vi "Day 24-Decomposed Instructions.vi"() -> ()   [LabVIEW 2021]
panel:
  out "Numeric":u64
  out "Model Number":u64
  in  "Input File":enum32{"example input", "input"}(radio)
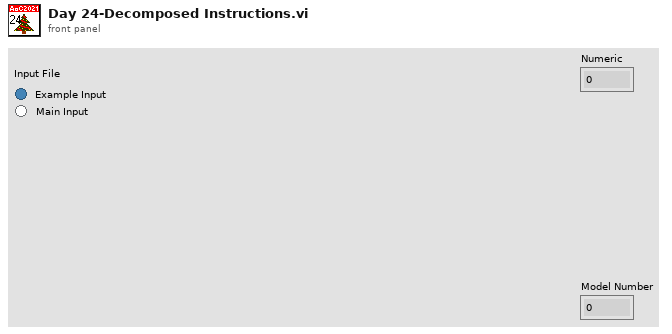
[diagram p1: front panel]
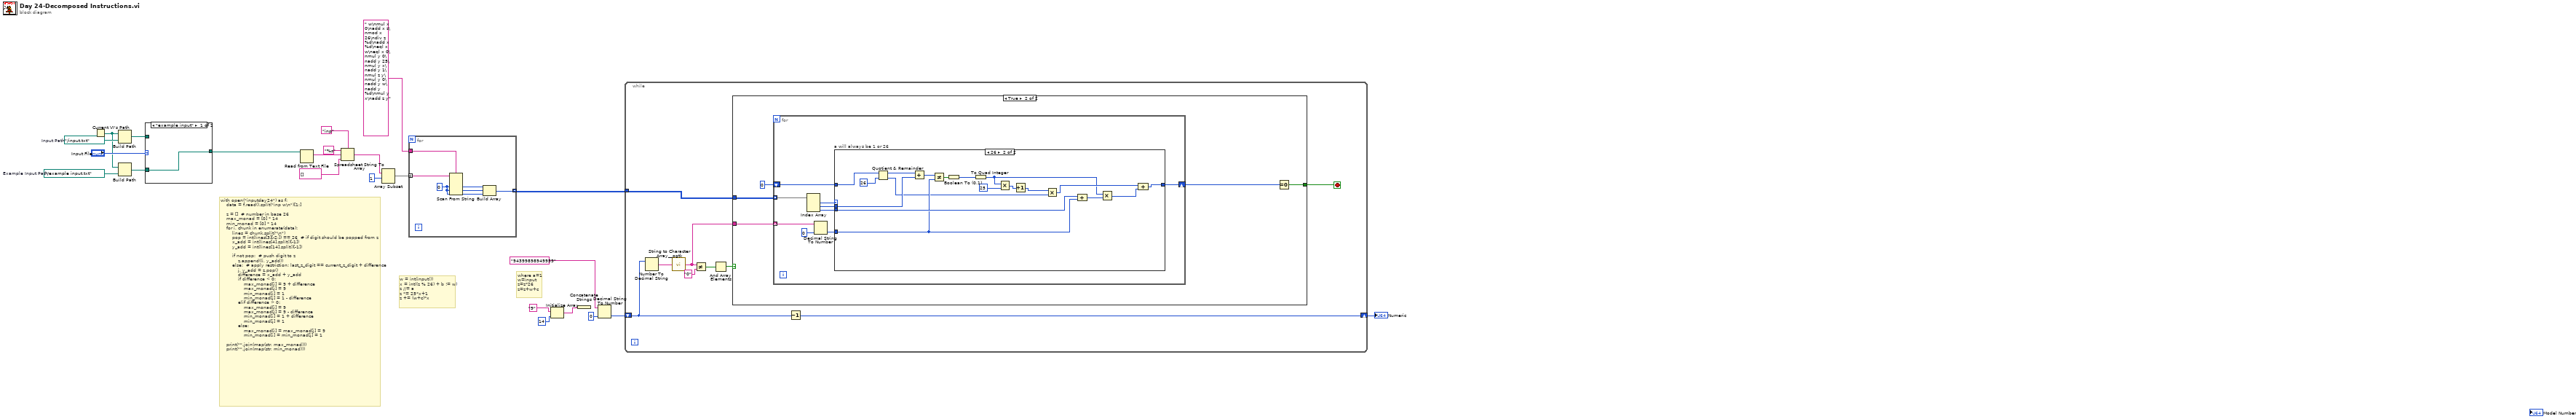
[diagram p0: block diagram]
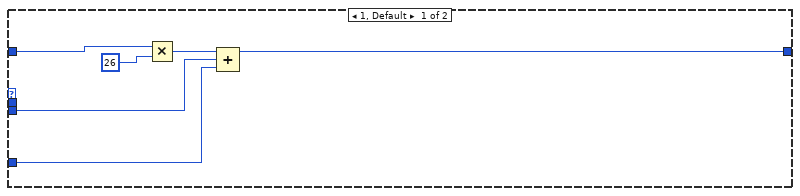
[diagram p4: hidden frame]
diagram:
  w22 = path "../example input.txt"  # Example Input Path
  w23 = path "../input.txt"  # Input Path
  # "with open(\"inputday24\") as f:\n    data = f.read().split(\"inp w\\n\")[1:]\n\n    z = []  # number in base 26\n    max_monad = [0] * 14\n    min_monad = [0] * 14\n    for i, chunk in enumerate(data):\n        lines = chunk.split(\"\\n\")\n        pop = int(lines[3][-2:]) == 26  # if digit should be popped from z\n        x_add = int(lines[4].split()[-1])\n        y_add = int(lines[14].split()[-1])\n\n        if not pop:  # push digit to z\n            z.append((i, y_add))\n        else:  # apply restriction: last_z_digit == current_z_digit + difference\n            j, y_add = z.pop()\n            difference = x_add + y_add\n            if difference < 0:\n                max_monad[i] = 9 + difference\n                max_monad[j] = 9\n                min_monad[i] = 1\n                min_monad[j] = 1 - difference\n            elif difference > 0:\n                max_monad[i] = 9\n                max_monad[j] = 9 - difference\n                min_monad[i] = 1 + difference\n                min_monad[j] = 1\n            else:\n                max_monad[i] = max_monad[j] = 9\n                min_monad[i] = min_monad[j] = 1\n\n    print(\"\".join(map(str, max_monad)))\n    print(\"\".join(map(str, min_monad)))"
  # "w = int(input())\nx = int((z % 26) + b != w)\nz //= a\nz *= 25*x+1\nz += (w+c)*x"
  # "where a=1\nw=input\nz=z*26\nz=z+w+c"
  n1 = Current VI's Path() -> (path=w18:path)
  n2 = Build Path(base path=w18, name or relative path=w23) -> (appended path=w20:path)
  n3 = Build Path(base path=w18, name or relative path=w22) -> (appended path=w19:path)
  n4 = case shown="\"example input\"" "Input File" {
    tunnel: w20 -> [_ w25]
    tunnel: w19 -> [w24 _]
    tunnel: [w24 w25] -> w17
    frame "example input" {
    }
    frame "input" {
    }
  }
  n5 = Read from Text File(file (use dialog)=w17) -> (text=w16:string)  [unwired: 3 in, 3 out]
  n6 = Spreadsheet String To Array(delimiter (Tab)="inp", format string="%s", spreadsheet string=w16, array type (2D Dbl)=string[] []) -> (array=w12:string[])
  n7 = Array Subset(array=w12, index=1) -> (w10:string[])  [unwired: 1 in]
  n8 = for {
    tunnel: w10 -> [w32] mode=indexing
    tunnel: " w\nmul x 0\nadd x z\nmod x 26\ndiv z %d\nadd x %d\neql x w\neql x 0\nmul y 0\nadd y 25\nmul y x\nadd y 1\nmul z y\nmul y 0\nadd y w\nadd y %d\nmul y x\nadd z y" -> [w31]
    tunnel: [w26] -> w8 mode=indexing
    w30 = i64 0 ("default value 1")
    n9 = Scan From String(format string=w31, input string=w32, default 1=w30, default 2=w30, default 3=w30) -> (output 1=w29:i64, output 2=w28:i64, output 3=w27:i64)  [unwired: 2 in, 3 out]
    n10 = Build Array(w29, w28, w27) -> (w26:i64[])
  }
  n11 = Initialize Array("9", 14) -> (w2:string[])
  n12 = Concatenate Strings(w2) -> ()  [unwired: 1 out]
  n13 = Decimal String To Number(string="94399898949959", default (0L)=u64 0 ("default (0 I32)")) -> (number=w6:u64)  [unwired: 1 in, 1 out]
  n14 = while {
    tunnel: w8 -> [w41]
    shift-right: [w40] -> w5
    shift-left: w6 -> [w36]
    stop <- w33 stop-if-true
    n15 = Number To Decimal String(number=w36) -> (decimal integer string=w38:string)  [unwired: 1 in]
    n16 = call <userlib>:"String to Character Array__ogtk.vi"("Input String"=w38) -> ("Character Array"=w34:string[])
    n17 = Not Equal?(x=w34, y="0") -> (x != y?=w37:bool[])
    n18 = And Array Elements(Boolean array=w37) -> (logical AND=w35:bool)
    n19 = case shown="True" w35 {
      tunnel: w41 -> [_ w45]
      tunnel: w34 -> [_ w44]
      tunnel: [_ w46] -> w33
      frame False {
      }
      frame True {
        n20 = for {
          tunnel: w45 -> [w49] mode=indexing
          tunnel: w44 -> [w48] mode=indexing
          shift-right: [w50] -> w43
          shift-left: i64 0 ("dimension size") -> [w47]
          n21 = Index Array(array=w49) -> (element #1=w52:i64, element #2=w53:i64, element #3=w51:i64)  [unwired: 3 in]
          n22 = Decimal String To Number(string=w48, default (0L)=i64 0 ("default (0 I32)")) -> (number=w55:i64)  [unwired: 1 in, 1 out]
          n23 = case "a will always be 1 or 26" shown="26" w52 {
            tunnel: w47 -> [w61 w73]
            tunnel: [w58 w63] -> w50
            tunnel: w51 -> [w57 w79]
            tunnel: w53 -> [_ w77]
            tunnel: w55 -> [w56 w69]
            frame 1, Default {
              n24 = Multiply(x=w61, y=i64 26) -> (x*y=w59:i64)
              n25 = Compound Arithmetic op=ADD(w59, w57, w56) -> (w58:i64)
            }
            frame 26 {
              n26 = Quotient & Remainder(x=w73, y=i64 26) -> (x-y*floor(x/y)=w68:i64, floor(x/y)=w62:i64)
              n27 = Add(x=w68, y=w77) -> (x+y=w76:i64)
              n28 = Not Equal?(x=w76, y=w69) -> (x != y?=w75:bool)
              n29 = Boolean To (0,1)(Boolean=w75) -> (0, 1=w74:i16)
              n30 = To Quad Integer(1:w74) -> (0:w65:i64)
              n31 = Multiply(x=w65, y=i64 25) -> (x*y=w70:i64)
              n32 = Increment(x=w70) -> (x+1=w72:i64)
              n33 = Multiply(x=w72, y=w62) -> (x*y=w67:i64)
              n34 = Compound Arithmetic op=ADD(w79, w69) -> (w66:i64)
              n35 = Multiply(x=w65, y=w66) -> (x*y=w64:i64)
              n36 = Compound Arithmetic op=ADD(w67, w64) -> (w63:i64)
            }
          }
        }
        n37 = Equal To 0?(x=w43) -> (x = 0?=w46:bool)
      }
    }
    n38 = Decrement(x=w36) -> (x-1=w40:u64)
  }
  "Numeric" <- w5
